vi "test Inhibit Bus A - Dual RT.vi"(8 "error in (no error)":errorcluster, 11 "RT Inhibit Bus A in":refnum<class "RT Inhibit Bus A.lvclass">) -> (0 "error out":errorcluster, 3 "RT Inhibit Bus A out":refnum<class "RT Inhibit Bus A.lvclass">)   [LabVIEW 2016, in "RT Inhibit Bus A.lvclass"]
uses:
  RT Inhibit Bus A.lvclass
  1553 Board/1553 Board.lvclass
  1553 Component/1553 Component.lvclass
  Remote Terminal/Remote Terminal.lvclass
  Remote Terminal/TypeDefs/RT Configuration.ctl
  1553 SubComponent/TypeDefs/Scaling Information.ctl
  1553 SubComponent/1553 SubComponent.lvclass
  1553 SubComponent/TypeDefs/Parameter Table Data.ctl
  Remote Terminal/TypeDefs/Command Type.ctl
  Remote Terminal/TypeDefs/Command Configuration.ctl
  PPLs/FPGA Interface.lvlibp/FPGA Interface/FPGA Interface.lvclass
  D:/SVN/Products/BCI-1553/Software/Development/2016/RealTime/1553 SubComponent/1553 SubComponent.lvclass
  Utilities/FPGA Interface/FPGA Interface.lvclass
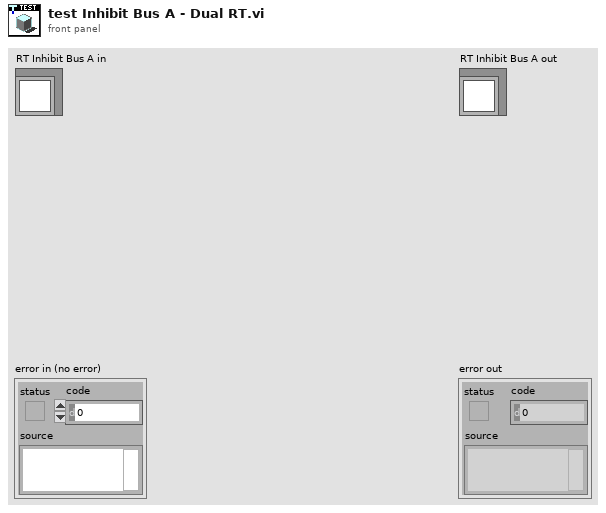
[diagram p1: front panel]
types:
  T1 = typedef "BCI-1553 API.lvlib/Remote Terminal.lvclass/Command Configuration.ctl" = cluster{"Command Type":T2, "Mode Code ID (1-32)":u16, "SubAddress (1-30)":u16, "Word Count (1-32)":u16, "Illegal Command":bool, "Broadcast":bool, "Data":u16[], "Data Fields":T3[]}
  T2 = typedef "BCI-1553 API.lvlib/Remote Terminal.lvclass/Command Type.ctl" = enum16{"Transmit", "Receive", "Mode Code Tx", "Mode Code Rx"}
  T3 = typedef "BCI-1553 API.lvlib/1553 SubComponent.lvclass/Parameter Table Data.ctl" = cluster{"Parameter Name":string, "Base Word":u16, "Address":u16, "Value":u64, "Mask":u16[], "Scaling Info":T4}
  T4 = typedef "BCI-1553 API.lvlib/1553 SubComponent.lvclass/Scaling Information.ctl" = cluster{"Bit Offset":i32, "Bit Count":i32, "LSB Resolution":dbl, "2's Complement":bool, "Big Endian":bool, "Sign Bit":bool}
  T5 = typedef "BCI-1553 API.lvlib/Remote Terminal.lvclass/RT Configuration.ctl" = cluster{"RT-RT TimeOut (us)":u8, "Inhibit Bus A":bool, "Inhibit Bus B":bool, "Broadcast CMD Invalid":bool, "UnDef MCs Invalid":bool, "Notice 2 Data Storage":bool, "SMCP":bool, "Temp RX Buffer":bool, "Alt BIT Enable":bool, "Auto Bus Shutdown":bool, "MC 17 Sync":u8, "MC 16 SR Reset":bool, "MC 8 Reset":bool}
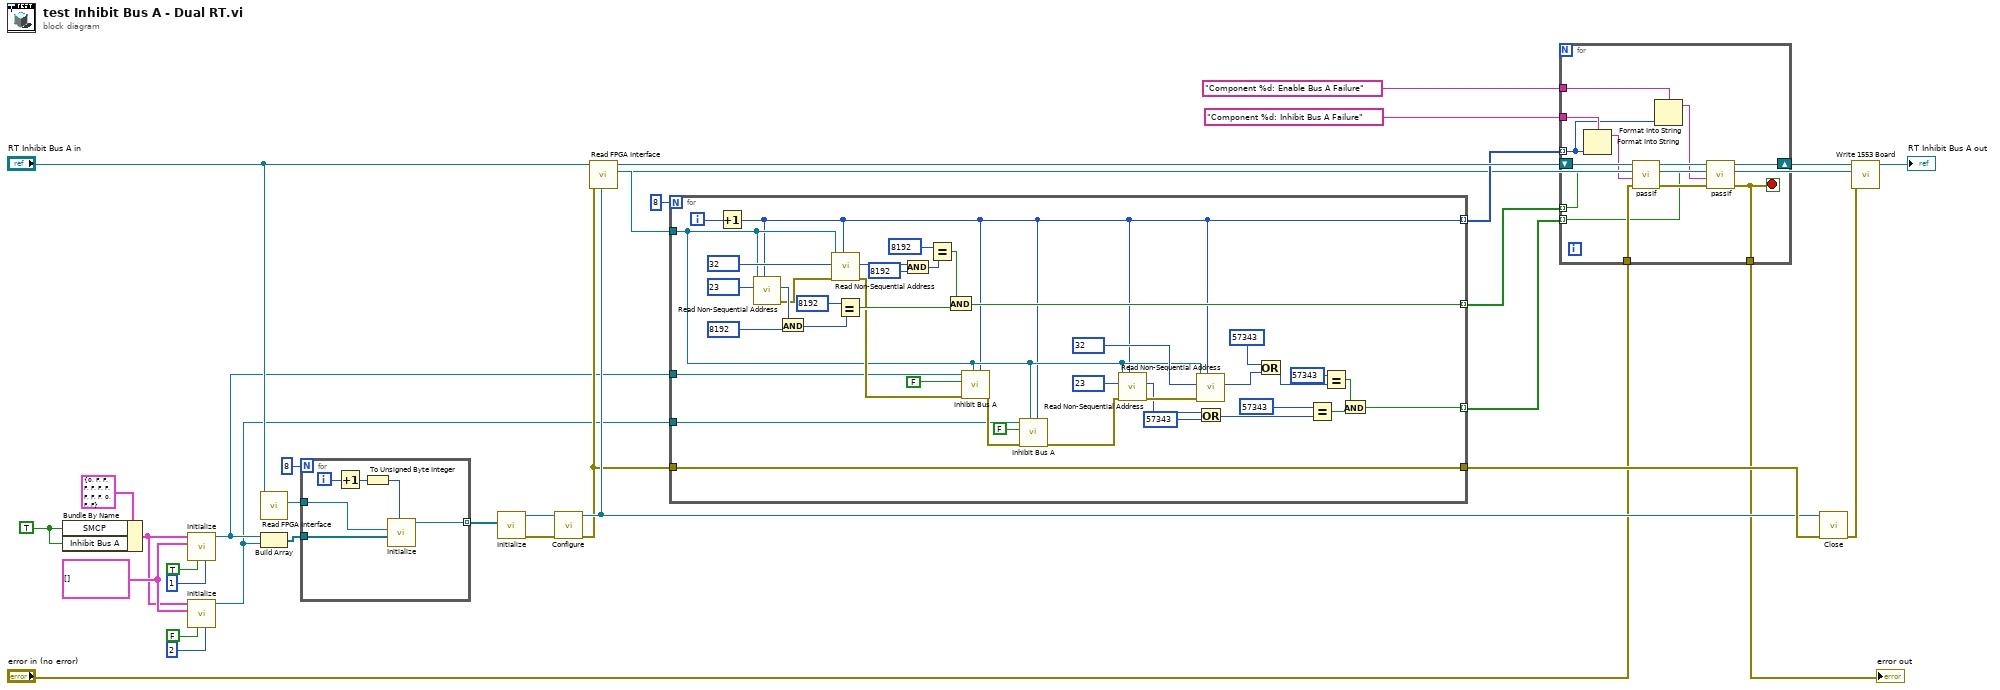
[diagram p0: block diagram]
diagram:
  w10 = T1[] [] ("Commands")
  w26 = TRUE ("SMCP")
  n1 = Bundle By Name(cluster=T5 {"RT-RT TimeOut (us)"=0, "Inhibit Bus A"=FALSE, "Inhibit Bus B"=FALSE, "Broadcast CMD Invalid"=FALSE, "UnDef MCs Invalid"=FALSE, "Notice 2 Data Storage"=FALSE, "SMCP"=FALSE, "Temp RX Buffer"=FALSE, "Alt BIT Enable"=FALSE, "Auto Bus Shutdown"=FALSE, "MC 17 Sync"=0, "MC 16 SR Reset"=FALSE, "MC 8 Reset"=FALSE} ("RT Configuration"), "SMCP"=w26, "Inhibit Bus A"=w26) -> (w9:T5)
  n2 = call "Initialize.vi"("RT Address (0-30)"=u8 1, "RT 1?"=TRUE, "Commands"=w10, "RT Configuration"=w9) -> ("Remote Terminal out"=w4:refnum<class "Remote Terminal.lvclass">)  [unwired: 6 in, 1 out]
  n3 = call "Initialize.vi"("RT Address (0-30)"=u8 2, "RT 1?"=FALSE, "Commands"=w10, "RT Configuration"=w9) -> ("Remote Terminal out"=w3:refnum<class "Remote Terminal.lvclass">)  [unwired: 6 in, 1 out]
  n4 = call-dynamic "Read FPGA Interface.vi"("1553 Test in"="RT Inhibit Bus A in") -> ("FPGA Interface"=w30:refnum<class "FPGA Interface.lvclass">)  [unwired: 8 in, 2 out]
  n5 = Build Array(w4, w3) -> (w31:refnum<class "Remote Terminal.lvclass">[])
  n6 = for {
    N: 8 -> [_]
    tunnel: [w37] -> w33 mode=indexing
    tunnel: w31 -> [w36]
    tunnel: w30 -> [w35]
    i -> [w39]
    n7 = Increment(x=w39) -> (x+1=w34:i32)
    n8 = To Unsigned Byte Integer(number=w34) -> (unsigned 8bit integer=w38:u8)
    n9 = call "Initialize.vi"("Component ID (1-8)"=w38, "SubComponents"=w36, "FPGA Interface"=w35) -> ("1553 Component out"=w37:refnum<class "1553 Component.lvclass">)  [unwired: 7 in, 1 out]
  }
  n10 = call "Initialize.vi"("Components"=w33) -> ("error out"=w15:errorcluster, "1553 Board out"=w17:refnum<class "1553 Board.lvclass">)  [unwired: 9 in]
  n11 = call-dynamic "Configure.vi"("error in (no error)"=w15, "1553 Board in"=w17) -> ("error out"=w14:errorcluster, "1553 Board out"=w16:refnum<class "1553 Board.lvclass">)  [unwired: 8 in]
  n12 = call-dynamic "Read FPGA Interface.vi"("error in (no error)"=w14, "1553 Test in"="RT Inhibit Bus A in") -> ("FPGA Interface"=w23:refnum<class "FPGA Interface.lvclass">, "1553 Test out"=w22:refnum<class "RT Inhibit Bus A.lvclass">)  [unwired: 7 in, 1 out]
  n13 = for {
    N: 8 -> [_]
    tunnel: w14 -> [w73]
    tunnel: [w73] -> w24
    tunnel: w23 -> [w54]
    tunnel: [w67] -> w20 mode=indexing
    tunnel: [w46] -> w19 mode=indexing
    tunnel: w4 -> [w49]
    tunnel: w3 -> [w48]
    tunnel: [w47] -> w1 mode=indexing
    i -> [w74]
    n14 = Increment(x=w74) -> (x+1=w46:i32)
    n15 = call-dynamic "Read Non-Sequential Address.vi"("Target IC (1-8)"=w46, "Address"=u16 23, "FPGA Interface in"=w54) -> ("error out"=w63:errorcluster, "Data"=w75:u16)  [unwired: 7 in]
    n16 = And(x=w75, y=u16 8192) -> (x .and. y?=w66:u16)
    n17 = call-dynamic "Read Non-Sequential Address.vi"("Target IC (1-8)"=w46, "error in (no error)"=w63, "Address"=u16 32, "FPGA Interface in"=w54) -> ("error out"=w55:errorcluster, "Data"=w64:u16)  [unwired: 6 in]
    n18 = Equal?(x=u16 8192, y=w66) -> (x = y?=w68:bool)
    n19 = And(x=w64, y=u16 8192) -> (x .and. y?=w65:u16)
    n20 = Equal?(x=u16 8192, y=w65) -> (x = y?=w69:bool)
    n21 = And(x=w69, y=w68) -> (x .and. y?=w67:bool)
    n22 = call-dynamic "Inhibit Bus A.vi"("Component ID"=w46, "FPGA Interface"=w54, "error in (no error)"=w55, "Inhibit Bus A?"=FALSE ("Bus B Inhibited?"), "Remote Terminal in"=w49) -> ("error out"=w53:errorcluster)  [unwired: 5 in, 1 out]
    n23 = call-dynamic "Inhibit Bus A.vi"("Component ID"=w46, "FPGA Interface"=w54, "error in (no error)"=w53, "Inhibit Bus A?"=FALSE ("Bus B Inhibited?"), "Remote Terminal in"=w48) -> ("error out"=w50:errorcluster)  [unwired: 5 in, 1 out]
    n24 = call-dynamic "Read Non-Sequential Address.vi"("Target IC (1-8)"=w46, "error in (no error)"=w50, "Address"=u16 23, "FPGA Interface in"=w54) -> ("error out"=w56:errorcluster, "Data"=w44:u16)  [unwired: 6 in]
    n25 = call-dynamic "Read Non-Sequential Address.vi"("Target IC (1-8)"=w46, "error in (no error)"=w56, "Address"=u16 32, "FPGA Interface in"=w54) -> ("Data"=w42:u16)  [unwired: 6 in, 1 out]
    n26 = Or(x=w44, y=u16 57343) -> (x .or. y?=w43:u16)
    n27 = Or(x=u16 57343, y=w42) -> (x .or. y?=w41:u16)
    n28 = Equal?(x=u16 57343, y=w43) -> (x = y?=w57:bool)
    n29 = Equal?(x=u16 57343, y=w41) -> (x = y?=w58:bool)
    n30 = And(x=w58, y=w57) -> (x .and. y?=w47:bool)
  }
  n31 = for {
    shift-right: [w83] -> w21
    shift-left: w22 -> [w91]
    tunnel: w20 -> [w90] mode=indexing
    tunnel: [w81] -> w7
    tunnel: "Component %d: Inhibit Bus A Failure" ("custom report message (\"\")") -> [w89]
    tunnel: w19 -> [w85] mode=indexing
    tunnel: "error in (no error)" -> [w87]
    tunnel: "Component %d: Enable Bus A Failure" ("custom report message (\"\")") -> [w86]
    tunnel: w1 -> [w80] mode=indexing
    stop <- w81 stop-if-true
    n32 = Format Into String(format string=w89, w85) -> (resulting string=w88:string)  [unwired: 2 in, 1 out]
    n33 = call-dynamic "passIf.vi"("error in (no error)"=w87, "message (\"\")"=w88, "pass"=w90, "TestCase in"=w91) -> ("error out"=w82:errorcluster, "TestCase out"=w84:refnum<class "RT Inhibit Bus A.lvclass">)  [unwired: 6 in]
    n34 = Format Into String(format string=w86, w85) -> (resulting string=w79:string)  [unwired: 2 in, 1 out]
    n35 = call-dynamic "passIf.vi"("error in (no error)"=w82, "message (\"\")"=w79, "pass"=w80, "TestCase in"=w84) -> ("error out"=w81:errorcluster, "TestCase out"=w83:refnum<class "RT Inhibit Bus A.lvclass">)  [unwired: 6 in]
  }
  "error out" <- w7
  n36 = call-dynamic "Close.vi"("error in (no error)"=w24, "1553 Board in"=w16) -> ("error out"=w25:errorcluster)  [unwired: 9 in]
  n37 = call-dynamic "Write 1553 Board.vi"("error in (no error)"=w25, "1553 Board"=w16, "1553 Test in"=w21) -> ("1553 Test out"=→"RT Inhibit Bus A out":refnum<class "RT Inhibit Bus A.lvclass">)  [unwired: 7 in, 1 out]
